vi "osciloscope_meas.vi"(7 "error in (no error)":errorcluster, 9 "Kalibracni bod":T1, 10 "VISA Refnum in":refnum<visa-resource-name>) -> (0 "error out":errorcluster, 1 "number":dbl, 2 "Raw data":string, 3 "VISA Refnum out":refnum<visa-resource-name>)   [LabVIEW 2022 SP3]
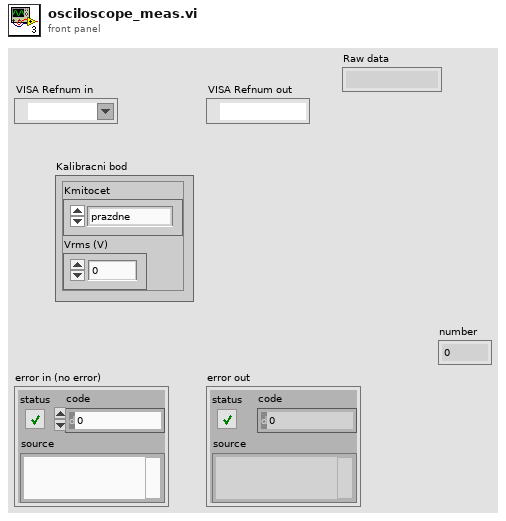
[diagram p1: front panel]
types:
  T1 = cluster{"Kmitocet":enum16{"prazdne", "50 Hz", "1 kHz", "5 kHz", "10 kHz", "20 kHz", "50 kHz", "100 kHz"}, "Vrms (V)":dbl}
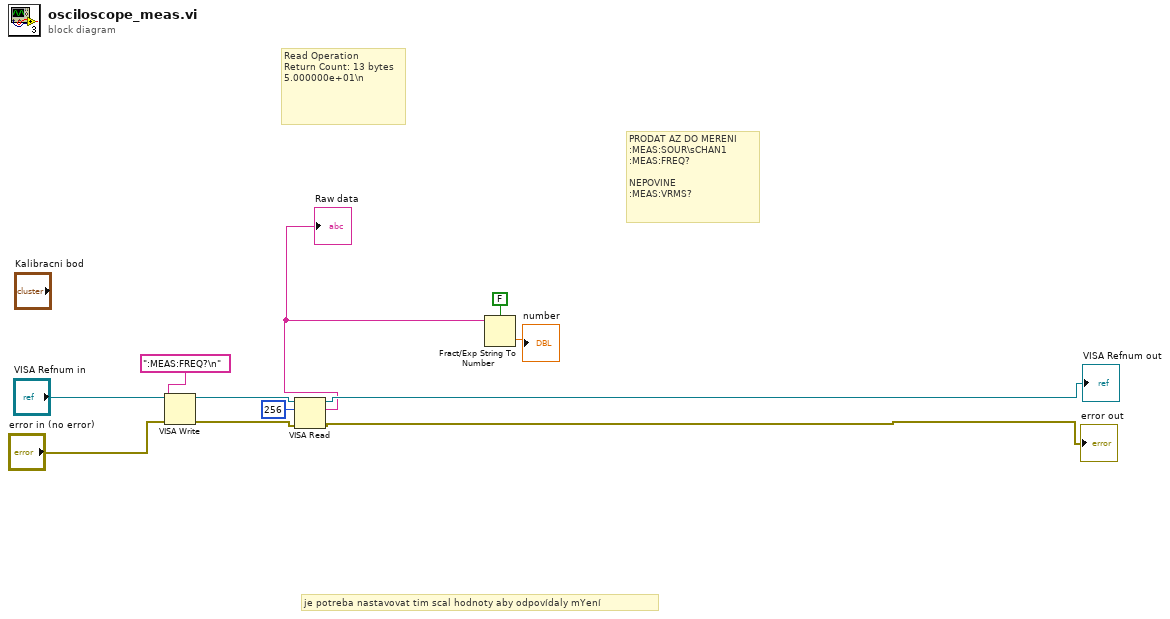
[diagram p0: block diagram]
diagram:
  # "Read Operation\nReturn Count: 13 bytes\n5.000000e+01\\n"
  # "je potreba nastavovat tim scal hodnoty aby odpovídaly mYení"
  # "PRODAT AZ DO MERENI\n:MEAS:SOUR\\sCHAN1\n:MEAS:FREQ?\n\nNEPOVINE\n:MEAS:VRMS?"
  n1 = VISA Write(VISA resource name="VISA Refnum in", write buffer=":MEAS:FREQ?\n", error in (no error)="error in (no error)") -> (VISA resource name out=w8:refnum<visa-resource-name>, error out=w7:errorcluster)  [unwired: 1 out]
  n2 = VISA Read(VISA resource name=w8, byte count=u32 256, error in (no error)=w7) -> (VISA resource name out=→"VISA Refnum out":refnum<visa-resource-name>, read buffer=w1:string, error out=→"error out":errorcluster)  [unwired: 1 out]
  "Raw data" <- w1
  n3 = Fract/Exp String To Number(use system decimal point (T)=FALSE, string=w1) -> (number=→"number":dbl)  [unwired: 2 in, 1 out]
